vi "Get Camera Position.vi"(9 "Distance":sgl, 10 "Longitude":sgl, 11 "Latitude":sgl) -> (3 "Camera Position":cluster{"X":sgl, "Y":sgl, "Z":sgl}={"X"=0.5, "Y"=0.5, "Z"=0.5})   [LabVIEW 2020, in "3D Plot.lvclass"]
uses:
  3D Plot.lvclass
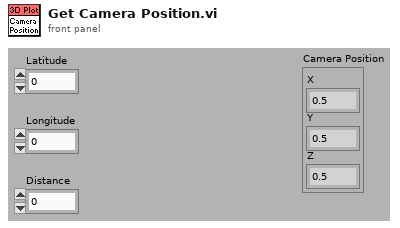
[diagram p1: front panel]
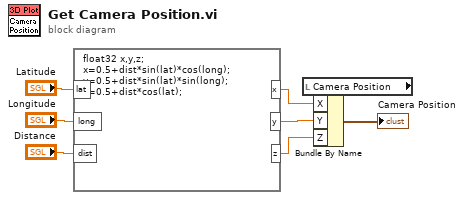
[diagram p0: block diagram]
diagram:
  n1 = formula code="float32 x,y,z;\nx=0.5+dist*sin(lat)*cos(long);\ny=0.5+dist*sin(lat)*sin(long);\nz=0.5+dist*cos(lat);"("lat"="Latitude", "long"="Longitude", "dist"="Distance") -> ("x"=w4:sgl, "y"=w3:sgl, "z"=w2:sgl)
  n2 = local read "Camera Position"() -> (w1:cluster{"X":sgl, "Y":sgl, "Z":sgl})
  n3 = Bundle By Name(cluster=w1, "X"=w4, "Y"=w3, "Z"=w2) -> (→"Camera Position":cluster{"X":sgl, "Y":sgl, "Z":sgl})
